vi "SiosIfmGetFilterSettings.vi"(0 "devNumber":i32) -> (1 "success":i32, 2 "FilterSettings":T1)   [LabVIEW 2009]
uses:
  siosifm.dll
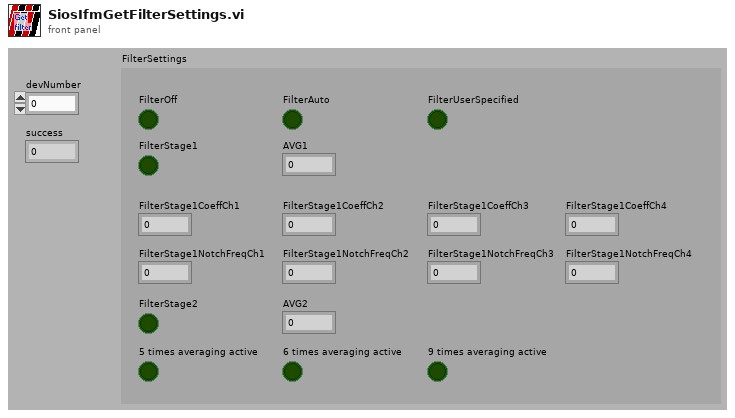
[diagram p1: front panel]
types:
  T1 = cluster{"FilterOff":bool, "FilterAuto":bool, "FilterUserSpecified":bool, "FilterStage1":bool, "AVG1":i32, "FilterStage1CoeffCh1":dbl, "FilterStage1CoeffCh2":dbl, "FilterStage1CoeffCh3":dbl, "FilterStage1CoeffCh4":dbl, "FilterStage1NotchFreqCh1":dbl, "FilterStage1NotchFreqCh2":dbl, "FilterStage1NotchFreqCh3":dbl, "FilterStage1NotchFreqCh4":dbl, "FilterStage2":bool, "AVG2":i32, "5 times averaging active":bool, "6 times averaging active":bool, "9 times averaging active":bool}
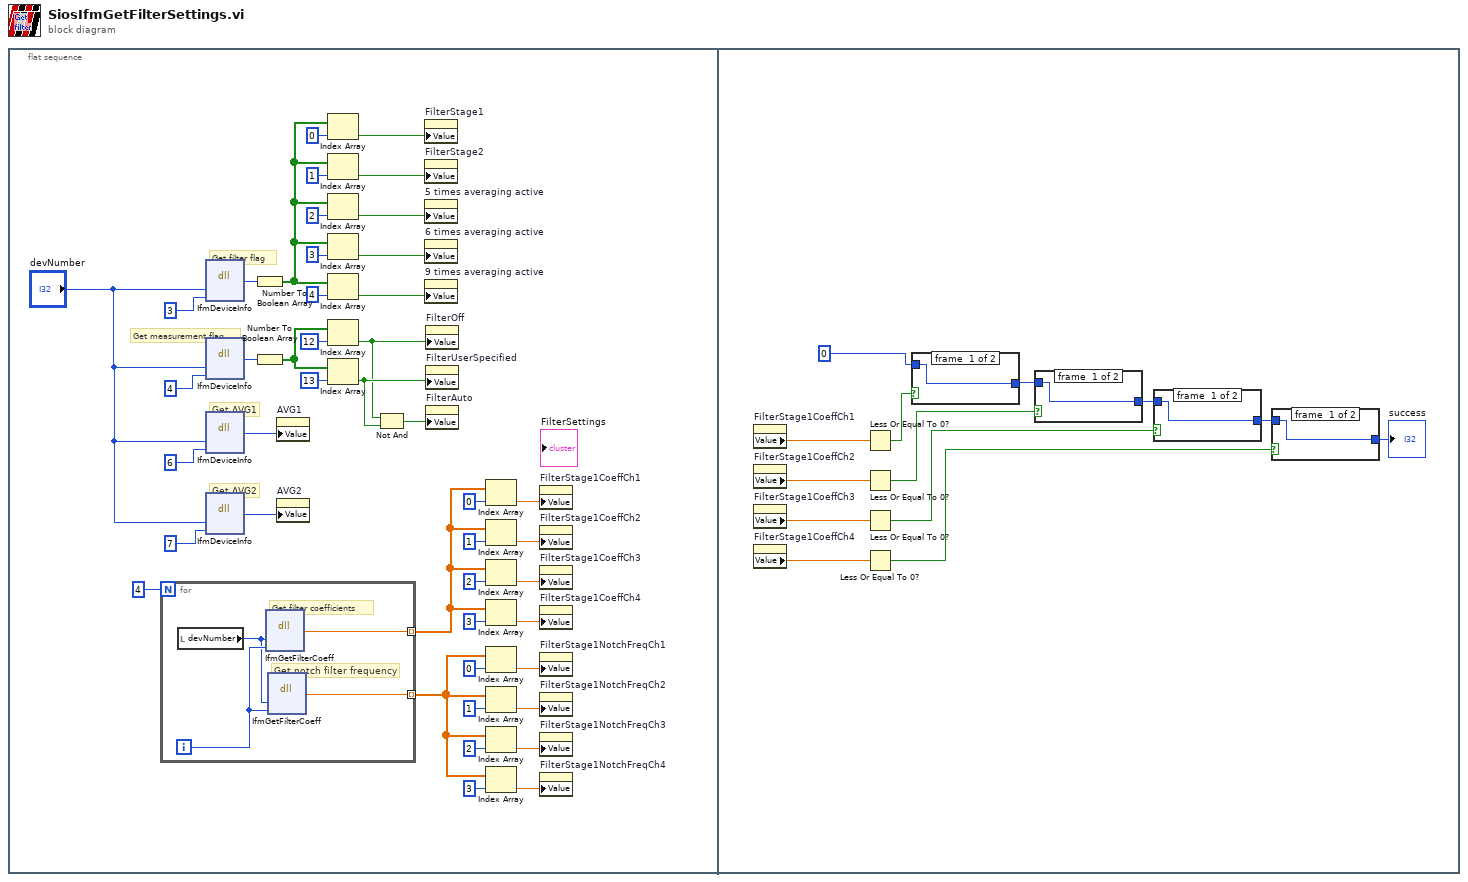
[diagram p0: block diagram]
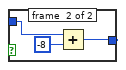
[diagram p2: hidden frame]
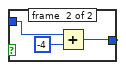
[diagram p3: hidden frame]
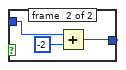
[diagram p4: hidden frame]
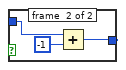
[diagram p5: hidden frame]
diagram:
  n1 = flat-sequence {
    frame #0 {
      # "Get AVG2"
      # "Get AVG1"
      # "Get measurement flag"
      # "Get filter flag"
      n2 = for {
        N: 4 -> [_]
        tunnel: [w47] -> w16 mode=indexing
        tunnel: [w46] -> w11 mode=indexing
        i -> [w49]
        # "Get notch filter frequency"
        # "Get filter coefficients"
        n3 = local read "devNumber"() -> (w48:i32)
        n4 = dll-call lib="D:/Support/Labview/RE-10/SIOS_IfmDLL/siosifm.dll" fn="IfmGetFilterCoeff"("devNumber"=w48, "channel"=w49) -> (w46:dbl)  [unwired: 5 in, 2 out]
        n5 = dll-call lib="D:/Support/Labview/RE-10/SIOS_IfmDLL/siosifm.dll" fn="IfmGetFilterCoeff"("devNumber"=w48, "channel"=w49) -> (w47:dbl)  [unwired: 5 in, 2 out]
      }
      n6 = dll-call lib="D:/Support/Labview/RE-10/SIOS_IfmDLL/siosifm.dll" fn="IfmDeviceInfo"("devNumber"="devNumber", "requestedInfoFlag"=u32 3) -> (w17:u32)  [unwired: 5 in, 2 out]
      n7 = dll-call lib="D:/Support/Labview/RE-10/SIOS_IfmDLL/siosifm.dll" fn="IfmDeviceInfo"("devNumber"="devNumber", "requestedInfoFlag"=u32 4) -> (w18:u32)  [unwired: 5 in, 2 out]
      n8 = dll-call lib="D:/Support/Labview/RE-10/SIOS_IfmDLL/siosifm.dll" fn="IfmDeviceInfo"("devNumber"="devNumber", "requestedInfoFlag"=u32 6) -> (w36:u32)  [unwired: 5 in, 2 out]
      n9 = dll-call lib="D:/Support/Labview/RE-10/SIOS_IfmDLL/siosifm.dll" fn="IfmDeviceInfo"("devNumber"="devNumber", "requestedInfoFlag"=u32 7) -> (w37:u32)  [unwired: 5 in, 2 out]
      n10 = Number To Boolean Array(number=w17) -> (Boolean array=w27:bool[])
      n11 = Number To Boolean Array(number=w18) -> (Boolean array=w21:bool[])
      n12 = property on="AVG1" class="DigitalWert (strikt)"("Value"=w36) -> ()  [unwired: 2 in, 2 out]
      n13 = property on="AVG2" class="DigitalWert (strikt)"("Value"=w37) -> ()  [unwired: 2 in, 2 out]
      n14 = Index Array(array=w27, index=0 ("Index")) -> (element=w32:bool)
      n15 = Index Array(array=w27, index=1 ("Index")) -> (element=w31:bool)
      n16 = Index Array(array=w27, index=2 ("Index")) -> (element=w30:bool)
      n17 = Index Array(array=w27, index=3 ("Index")) -> (element=w29:bool)
      n18 = Index Array(array=w27, index=4 ("Index")) -> (element=w28:bool)
      n19 = Index Array(array=w21, index=12 ("Index")) -> (element=w33:bool)
      n20 = Index Array(array=w21, index=13 ("Index")) -> (element=w34:bool)
      n21 = Not And(1:w34, 2:w33) -> (0:w35:bool)
      n22 = property on="FilterStage1" class="Boolesch (strikt)"("Value"=w32) -> ()  [unwired: 2 in, 2 out]
      n23 = property on="FilterStage2" class="Boolesch (strikt)"("Value"=w31) -> ()  [unwired: 2 in, 2 out]
      n24 = property on="5 times averaging active" class="Boolesch (strikt)"("Value"=w30) -> ()  [unwired: 2 in, 2 out]
      n25 = property on="6 times averaging active" class="Boolesch (strikt)"("Value"=w29) -> ()  [unwired: 2 in, 2 out]
      n26 = property on="9 times averaging active" class="Boolesch (strikt)"("Value"=w28) -> ()  [unwired: 2 in, 2 out]
      n27 = property on="FilterOff" class="Boolesch (strikt)"("Value"=w33) -> ()  [unwired: 2 in, 2 out]
      n28 = property on="FilterUserSpecified" class="Boolesch (strikt)"("Value"=w34) -> ()  [unwired: 2 in, 2 out]
      n29 = property on="FilterAuto" class="Boolesch (strikt)"("Value"=w35) -> ()  [unwired: 2 in, 2 out]
      n30 = Index Array(array=w11, index=0 ("Index")) -> (element=w39:dbl)
      n31 = Index Array(array=w11, index=1 ("Index")) -> (element=w40:dbl)
      n32 = Index Array(array=w11, index=2 ("Index")) -> (element=w41:dbl)
      n33 = Index Array(array=w11, index=3 ("Index")) -> (element=w42:dbl)
      n34 = Index Array(array=w16, index=0 ("Index")) -> (element=w43:dbl)
      n35 = Index Array(array=w16, index=1 ("Index")) -> (element=w44:dbl)
      n36 = Index Array(array=w16, index=2 ("Index")) -> (element=w45:dbl)
      n37 = Index Array(array=w16, index=3 ("Index")) -> (element=w38:dbl)
      n38 = property on="FilterStage1CoeffCh1" class="DigitalWert (strikt)"("Value"=w39) -> ()  [unwired: 2 in, 2 out]
      n39 = property on="FilterStage1CoeffCh2" class="DigitalWert (strikt)"("Value"=w40) -> ()  [unwired: 2 in, 2 out]
      n40 = property on="FilterStage1CoeffCh3" class="DigitalWert (strikt)"("Value"=w41) -> ()  [unwired: 2 in, 2 out]
      n41 = property on="FilterStage1CoeffCh4" class="DigitalWert (strikt)"("Value"=w42) -> ()  [unwired: 2 in, 2 out]
      n42 = property on="FilterStage1NotchFreqCh1" class="DigitalWert (strikt)"("Value"=w43) -> ()  [unwired: 2 in, 2 out]
      n43 = property on="FilterStage1NotchFreqCh2" class="DigitalWert (strikt)"("Value"=w44) -> ()  [unwired: 2 in, 2 out]
      n44 = property on="FilterStage1NotchFreqCh3" class="DigitalWert (strikt)"("Value"=w45) -> ()  [unwired: 2 in, 2 out]
      n45 = property on="FilterStage1NotchFreqCh4" class="DigitalWert (strikt)"("Value"=w38) -> ()  [unwired: 2 in, 2 out]
    }
    frame #1 {
      n46 = property on="FilterStage1CoeffCh1" class="DigitalWert (strikt)"() -> ("Value"=w62:dbl)  [unwired: 2 in, 2 out]
      n47 = property on="FilterStage1CoeffCh2" class="DigitalWert (strikt)"() -> ("Value"=w61:dbl)  [unwired: 2 in, 2 out]
      n48 = property on="FilterStage1CoeffCh3" class="DigitalWert (strikt)"() -> ("Value"=w60:dbl)  [unwired: 2 in, 2 out]
      n49 = property on="FilterStage1CoeffCh4" class="DigitalWert (strikt)"() -> ("Value"=w59:dbl)  [unwired: 2 in, 2 out]
      n50 = Less Or Equal To 0?(x=w62) -> (x <= 0?=w58:bool)
      n51 = Less Or Equal To 0?(x=w61) -> (x <= 0?=w55:bool)
      n52 = Less Or Equal To 0?(x=w60) -> (x <= 0?=w53:bool)
      n53 = Less Or Equal To 0?(x=w59) -> (x <= 0?=w51:bool)
      n54 = case shown="True" w58 {
        tunnel: 0 -> [w75 w78]
        tunnel: [w75 w76] -> w56
        frame #0 {
        }
        frame #1 {
          n55 = Add(x=w78, y=-1) -> (x+y=w76:i32)
        }
      }
      n56 = case shown="True" w55 {
        tunnel: w56 -> [w71 w74]
        tunnel: [w71 w72] -> w54
        frame #0 {
        }
        frame #1 {
          n57 = Add(x=w74, y=-2) -> (x+y=w72:i32)
        }
      }
      n58 = case shown="True" w53 {
        tunnel: w54 -> [w67 w70]
        tunnel: [w67 w68] -> w52
        frame #0 {
        }
        frame #1 {
          n59 = Add(x=w70, y=-4) -> (x+y=w68:i32)
        }
      }
      n60 = case shown="True" w51 {
        tunnel: w52 -> [w63 w66]
        tunnel: [w63 w64] -> w50
        frame #0 {
        }
        frame #1 {
          n61 = Add(x=w66, y=-8) -> (x+y=w64:i32)
        }
      }
      "success" <- w50
    }
  }
